vi "AddTextToJPEGfile.vi"(6 "quality (80)":i32=80, 8 "error in (no error)":errorcluster, 9 "text":string, 10 "savePath":path, 11 "loadPath":path) -> (0 "error out":errorcluster, 2 "finalPath":path)   [LabVIEW 2021]
uses:
  TOAPspecs.ctl
  d31ad6ee-648f-a04d-8649-19cc048ae878.vi
panel:
  in  "TOAPspecs":T1={"textOrigin"={"x"=0, "y"=0}, "textAlignment"={"horizontal"=enum."left", "vertical"=enum."top"}, "fontColour"={"text color"=16448250, "BG color"=1132933, "orientation "=enum."None"}, "fontChoice"=enum."User-specified Font", "userFont"={"Font Name:"="Courier New", "Size"=36, "Strikeout?"=FALSE, "Italic?"=FALSE, "Underline?"=FALSE, "Outline?"=FALSE, "Shadow?"=FALSE, "Bold?"=FALSE}}
  out "2D Picture":picture
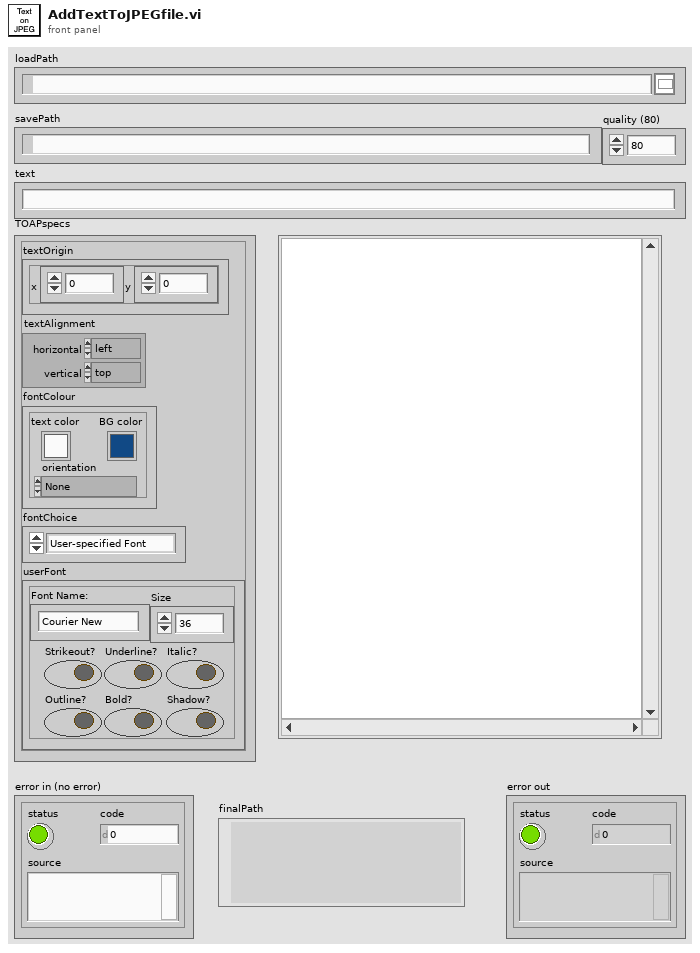
[diagram p1: front panel]
types:
  T1 = typedef "TOAPspecs.ctl" = cluster{"textOrigin":cluster{"x":i16, "y":i16}, "textAlignment":cluster{"horizontal":enum16{"left", "center", "right"}, "vertical":enum16{"top", "center", "bottom"}}, "fontColour":cluster{"text color":u32, "BG color":u32, "orientation ":enum16{"None", "Stacked", "Clockwise", "Counterclockwise"}}, "fontChoice":enum16{"User-specified Font", "Application Font", "System Font", "Dialog Font"}, "userFont":cluster{"Font Name:":string, "Size":i16, "Strikeout?":bool, "Italic?":bool, "Underline?":bool, "Outline?":bool, "Shadow?":bool, "Bold?":bool}}
  T2 = typedef "imagedata.ctl" = cluster{"image type":i32, "image depth":i32, "image":u8[], "mask":u8[], "colors":u32[], "Rectangle":cluster{"left":i16, "top":i16, "right":i16, "bottom":i16}}
  T3 = cluster{"Font Name:":string, "Size":i16, "Strikeout?":bool, "Italic?":bool, "Underline?":bool, "Outline?":bool, "Shadow?":bool, "Bold?":bool}
  T4 = enum16{"User-specified Font", "Application Font", "System Font", "Dialog Font"}
  T5 = cluster{"horizontal":enum16{"left", "center", "right"}, "vertical":enum16{"top", "center", "bottom"}}
  T6 = enum16{"None", "Stacked", "Clockwise", "Counterclockwise"}
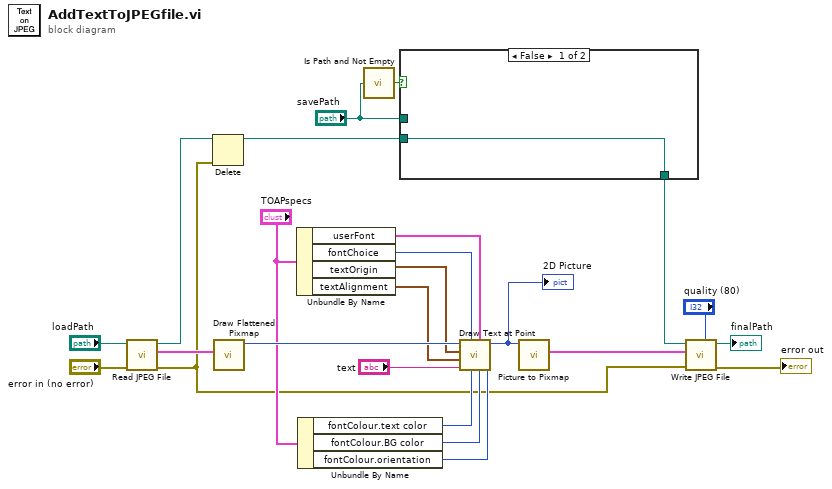
[diagram p0: block diagram]
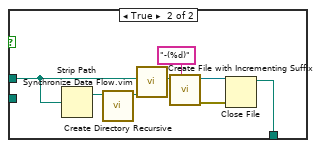
[diagram p2: hidden frame]
diagram:
  n1 = call <vilib>:"Read JPEG File.vi"("error in (no error)"="error in (no error)", "path to JPEG file"="loadPath") -> ("error out"=w7:errorcluster, "image data"=w18:T2, "path"=w4:path)  [unwired: 7 in]
  n2 = Delete(path (use dialog)=w4, error in=w7) -> (deleted path=w5:path)  [unwired: 3 in, 2 out]
  n3 = call <vilib>:"Draw Flattened Pixmap.vi"("image data"=w18) -> ("new picture"=w19:picture)  [unwired: 8 in]
  n4 = Unbundle By Name("TOAPspecs") -> ("userFont"=w14:T3, "fontChoice"=w13:T4, "textOrigin"=w12:cluster{"x":i16, "y":i16}, "textAlignment"=w11:T5)
  n5 = Unbundle By Name("TOAPspecs") -> ("fontColour.text color"=w10:u32, "fontColour.BG color"=w9:u32, "fontColour.orientation"=w8:T6)
  n6 = call <vilib>:"Is Path and Not Empty.vi"("path"="savePath") -> ("Is Path and Not Empty?"=w17:bool)  [unwired: 4 in]
  n7 = case shown="False" w17 {
    tunnel: "savePath" -> [_ w31]
    tunnel: w5 -> [w25 _]
    tunnel: [w25 w26] -> w3
    frame False {
    }
    frame True {
      n8 = Strip Path(path=w31) -> (stripped path=w32:path)  [unwired: 1 out]
      n9 = call <vilib>:"Create Directory Recursive.vi"("directory"=w32) -> ("directory copy"=w29:path)  [unwired: 4 in, 2 out]
      n10 = call "Synchronize Data Flow.vim"("input 4"=w29, "input 2"=w31) -> ("output 2"=w30:path)  [unwired: 2 in, 3 out]
      n11 = call <vilib>:"Create File with Incrementing Suffix.vi"("format string (\" (%d)\")"="-(%d)" ("format string (\" (%d)\")"), "file path"=w30) -> ("error out"=w27:errorcluster, "refnum out"=w28:refnum<file>)  [unwired: 7 in, 1 out]
      n12 = Close File(refnum=w28, error in=w27) -> (path=w26:path)  [unwired: 1 out]
    }
  }
  n13 = call <vilib>:"Draw Text at Point.vi"("text orientation"=w8, "BG color(transparent)"=w9, "[user-specified font]"=w14, "text color(black)"=w10, "desired font(Application)"=w13, "text"="text", "alignment(left, top)"=w11, "origin"=w12, "picture"=w19) -> ("new picture"=w21:picture)  [unwired: 1 in, 1 out]
  "2D Picture" <- w21
  n14 = call <vilib>:"Picture to Pixmap.vi"("picture"=w21) -> ("image data"=w22:T2)  [unwired: 9 in, 1 out]
  n15 = call <vilib>:"Write JPEG File.vi"("quality (80)"="quality (80)", "error in (no error)"=w7, "image data"=w22, "path to JPEG file"=w3) -> ("error out"=→"error out":errorcluster, "path"=→"finalPath":path)  [unwired: 6 in]
